vi "Get.vi"(7 "Binding":refnum<class "Binding.lvclass">, 8 "error in (no error)":errorcluster, 11 "Class in":refnum<class>) -> (0 "error out":errorcluster, 2 "Value":variant, 3 "Class out":refnum<class>)   [LabVIEW 2020, in "PropertyBinder.lvlib" / "Binding.lvclass"]
uses:
  Binding.lvclass
  Binding.lvclass/Binding.ctl
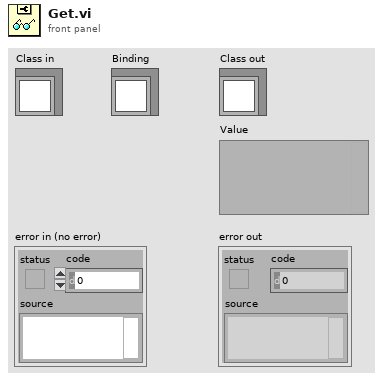
[diagram p1: front panel]
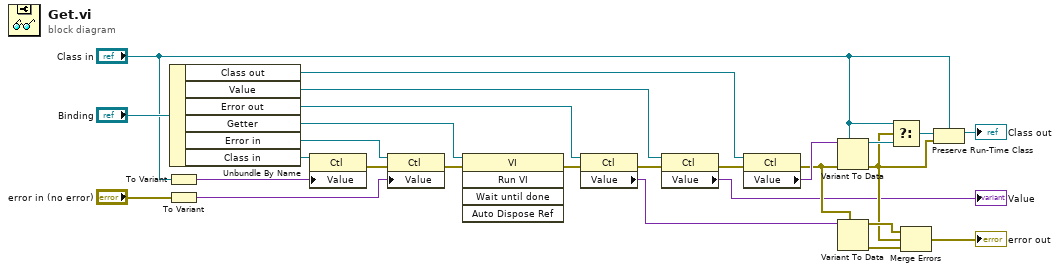
[diagram p0: block diagram]
diagram:
  n1 = To Variant(anything="Class in") -> (Variant=w22:variant)
  n2 = To Variant(anything="error in (no error)") -> (Variant=w20:variant)
  n3 = Unbundle By Name("Binding") -> ("Class out"=w11:refnum<vi>, "Value"=w4:refnum<vi>, "Error out"=w17:refnum<vi>, "Getter"=w24:refnum<vi>, "Error in"=w21:refnum<vi>, "Class in"=w23:refnum<vi>)
  n4 = property class="Ctl"(reference=w23, "Value"=w22) -> (error out=w7:errorcluster)  [unwired: 1 in, 1 out]
  n5 = property class="Ctl"(reference=w21, error in=w7, "Value"=w20) -> (error out=w19:errorcluster)  [unwired: 1 out]
  n6 = invoke class="VI" method="Run VI"(reference=w24, error in=w19) -> (error out=w18:errorcluster)  [unwired: 3 in, 4 out]
  n7 = property class="Ctl"(reference=w17, error in=w18) -> (error out=w6:errorcluster, "Value"=w16:variant)  [unwired: 1 out]
  n8 = property class="Ctl"(reference=w4, error in=w6) -> (error out=w5:errorcluster, "Value"=→"Value":variant)  [unwired: 1 out]
  n9 = property class="Ctl"(reference=w11, error in=w5) -> (error out=w12:errorcluster, "Value"=w13:variant)  [unwired: 1 out]
  n10 = Variant To Data(error in=w12, type="Class in", Variant=w13) -> (data=w26:refnum<class>, error out=w14:errorcluster)
  n11 = Variant To Data(type=w12, Variant=w16) -> (data=w15:errorcluster, error out=w27:errorcluster)  [unwired: 1 in]
  n12 = Select(t="Class in", s=w14, f=w26) -> (s? t:f=w25:refnum<class>)
  n13 = Merge Errors(w15, w14, w27) -> (→"error out":errorcluster)
  n14 = Preserve Run-Time Class(object in=w25, error in=w14, 2:"Class in") -> (object out=→"Class out":refnum<class>)  [unwired: 1 out]
